vi "ATF-Pump-Data queue.vi"(3 "error in":errorcluster) -> (7 "Data FIFO Ref":T1, 10 "error out":errorcluster)   [LabVIEW 2022 SP3]
uses:
  RT Controls/ATF-Pump-Data FIFO.ctl
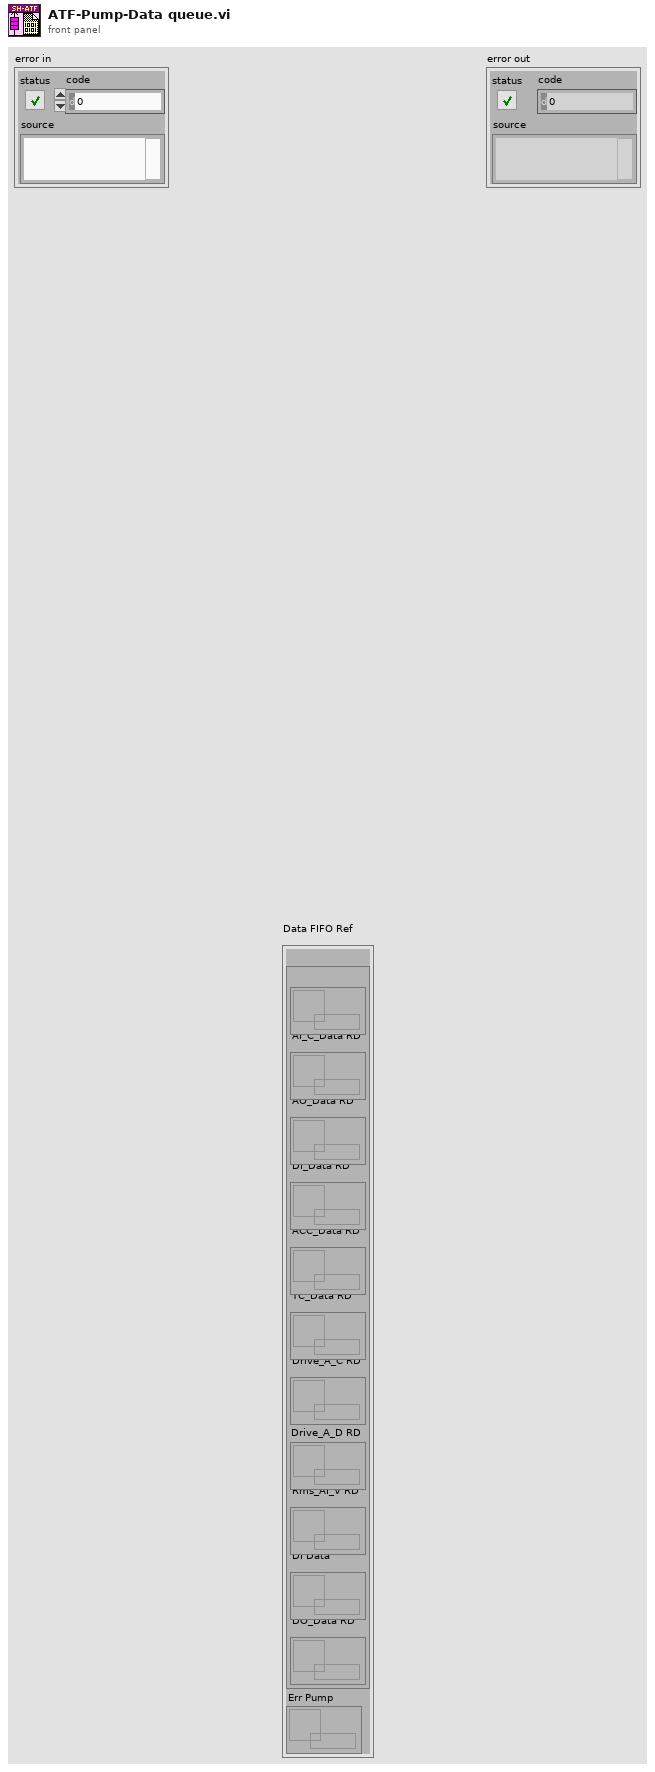
[diagram p1: front panel]
types:
  T1 = typedef "ATF-Pump-Data FIFO.ctl" = cluster{"RD":cluster{"AI_V_Data RD":refnum<queue>, "AI_C_Data RD":refnum<queue>, "AO_Data RD":refnum<queue>, "DI_Data RD":refnum<queue>, "ACC_Data RD":refnum<queue>, "TC_Data RD":refnum<queue>, "Drive_A_C RD":refnum<queue>, "Drive_A_D RD":refnum<queue>, "Rms_AI_V RD":refnum<queue>, "DI Data":refnum<queue>, "DO_Data RD":refnum<queue>}, "Err Pump":refnum<queue>}
  T2 = cluster{"AI_V_Data RD":refnum<queue>, "AI_C_Data RD":refnum<queue>, "AO_Data RD":refnum<queue>, "DI_Data RD":refnum<queue>, "ACC_Data RD":refnum<queue>, "TC_Data RD":refnum<queue>, "Drive_A_C RD":refnum<queue>, "Drive_A_D RD":refnum<queue>, "Rms_AI_V RD":refnum<queue>, "DI Data":refnum<queue>, "DO_Data RD":refnum<queue>}
  T3 = cluster{"Error Code":string, "Error Source":string}
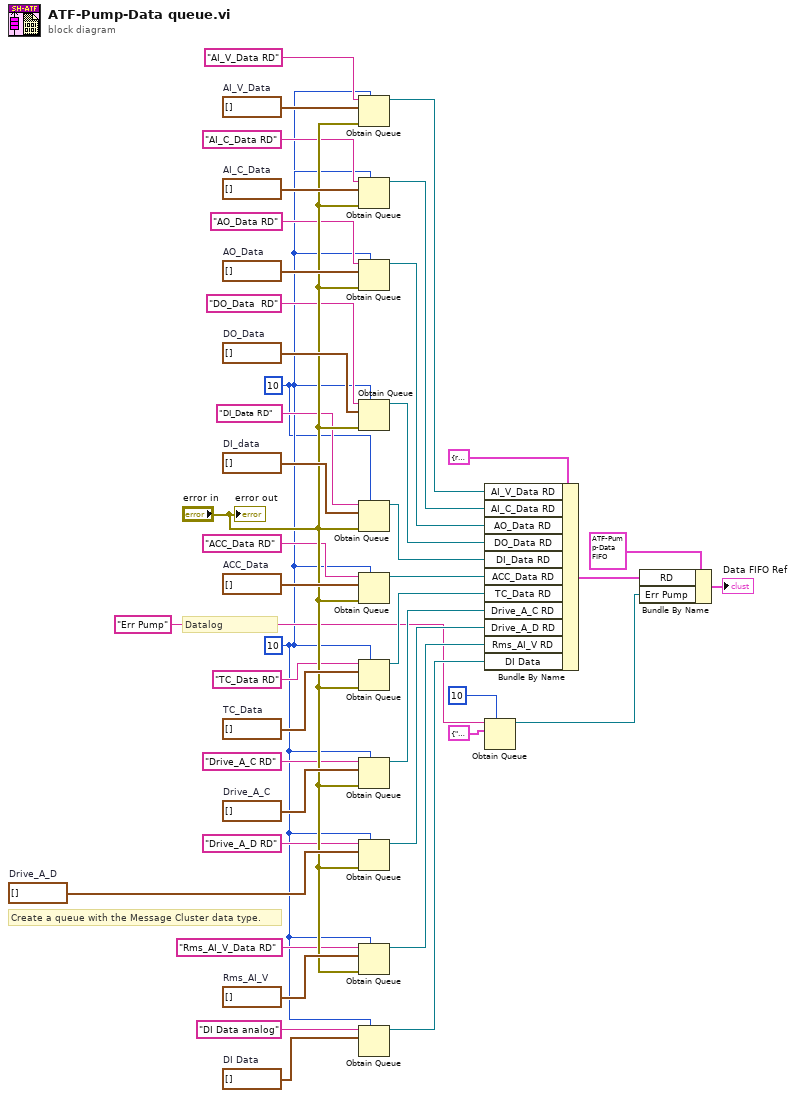
[diagram p0: block diagram]
diagram:
  w1 = 10 ("max queue size (-1, unlimited)")
  w11 = waveform(dbl)[] []  # DI Data
  w2 = 10 ("max queue size (-1, unlimited)")
  w44 = waveform(dbl)[] []  # AI_V_Data
  w35 = waveform(dbl)[] []  # Rms_AI_V
  w36 = waveform(dbl)[] []  # Drive_A_D
  w37 = waveform(dbl)[] []  # Drive_A_C
  w38 = waveform(dbl)[] []  # TC_Data
  w39 = waveform(dbl)[] []  # ACC_Data
  w41 = digitalwaveform[] []  # DI_data
  w40 = waveform(dbl)[] []  # DO_Data
  w42 = waveform(dbl)[] []  # AO_Data
  w43 = waveform(dbl)[] []  # AI_C_Data
  # "Create a queue with the Message Cluster data type."
  # "Datalog"
  n1 = Obtain Queue(max queue size (-1, unlimited)=w1, name (unnamed)="AI_V_Data RD", element data type=w44, error in (no error)="error in") -> (queue out=w34:refnum<queue>)  [unwired: 1 in, 2 out]
  n2 = Obtain Queue(max queue size (-1, unlimited)=w2, name (unnamed)="AI_C_Data RD", element data type=w43, error in (no error)="error in") -> (queue out=w33:refnum<queue>)  [unwired: 1 in, 2 out]
  n3 = Obtain Queue(max queue size (-1, unlimited)=w2, name (unnamed)="AO_Data RD", element data type=w42, error in (no error)="error in") -> (queue out=w32:refnum<queue>)  [unwired: 1 in, 2 out]
  n4 = Obtain Queue(max queue size (-1, unlimited)=w1, name (unnamed)="DO_Data  RD", element data type=w40, error in (no error)="error in") -> (queue out=w31:refnum<queue>)  [unwired: 1 in, 2 out]
  n5 = Obtain Queue(max queue size (-1, unlimited)=w1, name (unnamed)="DI_Data RD", element data type=w41, error in (no error)="error in") -> (queue out=w30:refnum<queue>)  [unwired: 1 in, 2 out]
  n6 = Obtain Queue(max queue size (-1, unlimited)=w2, name (unnamed)="ACC_Data RD", element data type=w39, error in (no error)="error in") -> (queue out=w29:refnum<queue>)  [unwired: 1 in, 2 out]
  n7 = Obtain Queue(max queue size (-1, unlimited)=w2, name (unnamed)="TC_Data RD", element data type=w38, error in (no error)="error in") -> (queue out=w28:refnum<queue>)  [unwired: 1 in, 2 out]
  n8 = Obtain Queue(max queue size (-1, unlimited)=w2, name (unnamed)="Drive_A_C RD", element data type=w37, error in (no error)="error in") -> (queue out=w27:refnum<queue>)  [unwired: 1 in, 2 out]
  n9 = Obtain Queue(max queue size (-1, unlimited)=w2, name (unnamed)="Drive_A_D RD", element data type=w36, error in (no error)="error in") -> (queue out=w26:refnum<queue>)  [unwired: 1 in, 2 out]
  n10 = Obtain Queue(max queue size (-1, unlimited)=w2, name (unnamed)="Rms_AI_V_Data RD", element data type=w35, error in (no error)="error in") -> (queue out=w25:refnum<queue>)  [unwired: 1 in, 2 out]
  n11 = Obtain Queue(max queue size (-1, unlimited)=w2, name (unnamed)="DI Data analog", element data type=w11) -> (queue out=w10:refnum<queue>)  [unwired: 2 in, 2 out]
  n12 = Bundle By Name(cluster=T2 {"AI_V_Data RD"=refnum, "AI_C_Data RD"=refnum, "AO_Data RD"=refnum, "DI_Data RD"=refnum, "ACC_Data RD"=refnum, "TC_Data RD"=refnum, "Drive_A_C RD"=refnum, "Drive_A_D RD"=refnum, "Rms_AI_V RD"=refnum, "DI Data"=refnum, "DO_Data RD"=refnum} ("RD"), "AI_V_Data RD"=w34, "AI_C_Data RD"=w33, "AO_Data RD"=w32, "DO_Data RD"=w31, "DI_Data RD"=w30, "ACC_Data RD"=w29, "TC_Data RD"=w28, "Drive_A_C RD"=w27, "Drive_A_D RD"=w26, "Rms_AI_V RD"=w25, "DI Data"=w10) -> (w3:T2)
  n13 = Obtain Queue(max queue size (-1, unlimited)=10, name (unnamed)="Err Pump", element data type=T3 {"Error Code"="", "Error Source"=""} ("element")) -> (queue out=w6:refnum<queue>)  [unwired: 2 in, 2 out]
  n14 = Bundle By Name(cluster=T1 {"RD"={"AI_V_Data RD"=refnum, "AI_C_Data RD"=refnum, "AO_Data RD"=refnum, "DI_Data RD"=refnum, "ACC_Data RD"=refnum, "TC_Data RD"=refnum, "Drive_A_C RD"=refnum, "Drive_A_D RD"=refnum, "Rms_AI_V RD"=refnum, "DI Data"=refnum, "DO_Data RD"=refnum}, "Err Pump"=refnum} ("Data FIFO Ref"), "RD"=w3, "Err Pump"=w6) -> (→"Data FIFO Ref":T1)
  "error out" <- "error in"
